vi "Less Than.vi"(9 "Semver 2":refnum<class "Semver.lvclass">, 10 "Semver 1":refnum<class "Semver.lvclass">) -> (2 "Version 1 < Version 2":bool)   [LabVIEW 2017, in "Semver.lvlib" / "Semver.lvclass"]
uses:
  Semver.lvclass
  Semver.lvclass/Semver.ctl
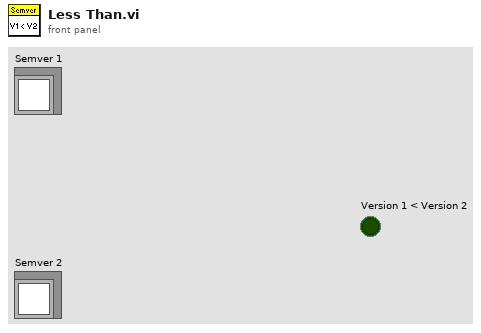
[diagram p1: front panel]
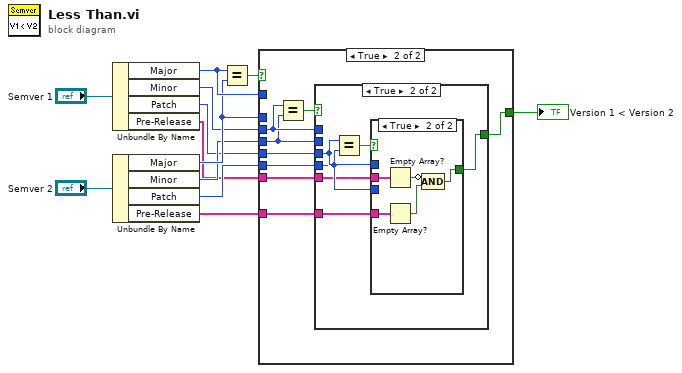
[diagram p0: block diagram]
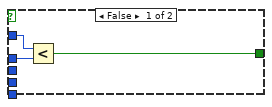
[diagram p2: hidden frame]
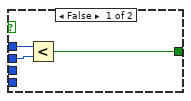
[diagram p3: hidden frame]
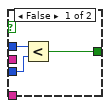
[diagram p4: hidden frame]
diagram:
  n1 = Unbundle By Name("Semver 1") -> ("Major"=w11:i32, "Minor"=w9:i32, "Patch"=w7:i32, "Pre-Release"=w5:string[])
  n2 = Unbundle By Name("Semver 2") -> ("Major"=w10:i32, "Minor"=w8:i32, "Patch"=w6:i32, "Pre-Release"=w4:string[])
  n3 = Equal?(x=w11, y=w10) -> (x = y?=w12:bool)
  n4 = case shown="True" w12 {
    tunnel: w11 -> [w15 _]
    tunnel: w10 -> [w14 _]
    tunnel: [w13 w20] -> w1
    tunnel: w9 -> [_ w22]
    tunnel: w8 -> [_ w21]
    tunnel: w7 -> [_ w19]
    tunnel: w6 -> [_ w18]
    tunnel: w5 -> [_ w17]
    tunnel: w4 -> [_ w16]
    frame False {
      n5 = Less?(x=w15, y=w14) -> (x < y?=w13:bool)
    }
    frame True {
      n6 = Equal?(x=w22, y=w21) -> (x = y?=w23:bool)
      n7 = case shown="True" w23 {
        tunnel: w22 -> [w26 _]
        tunnel: w21 -> [w25 _]
        tunnel: [w24 w29] -> w20
        tunnel: w19 -> [_ w31]
        tunnel: w18 -> [_ w30]
        tunnel: w17 -> [_ w28]
        tunnel: w16 -> [_ w27]
        frame False {
          n8 = Less?(x=w26, y=w25) -> (x < y?=w24:bool)
        }
        frame True {
          n9 = Equal?(x=w31, y=w30) -> (x = y?=w32:bool)
          n10 = case shown="True" w32 {
            tunnel: w31 -> [w35 _]
            tunnel: w30 -> [w34 _]
            tunnel: [w33 w36] -> w29
            tunnel: w28 -> [_ w40]
            tunnel: w27 -> [_ w39]
            frame False {
              n11 = Less?(x=w35, y=w34) -> (x < y?=w33:bool)
            }
            frame True {
              n12 = Empty Array?(array=w40) -> (empty?=w38:bool)
              n13 = Empty Array?(array=w39) -> (empty?=w37:bool)
              n14 = Compound Arithmetic op=AND(invert w38, w37) -> (w36:bool)
            }
          }
        }
      }
    }
  }
  "Version 1 < Version 2" <- w1
